vi "IMAQWriteMultiMetadata.vi"(0 "GRMActor in":refnum<class "GenericActor.lvclass">, 5 "Image In":T1, 7 "Keys":string[](array[string]), 9 "Values":dbl[](array[numeric]), 11 "error in (no error)":errorcluster, 12 "precision (6)":i16) -> (4 "GRMActor out":refnum<class "GenericActor.lvclass">, 6 "Image Out":T1, 15 "error out":errorcluster)   [LabVIEW 2020, in "GenericActor.lvlib" / "GenericActor.lvclass"]
uses:
  GenericActor.lvclass
  <vilib>/vision/Image Controls.llb/IMAQ Image.ctl
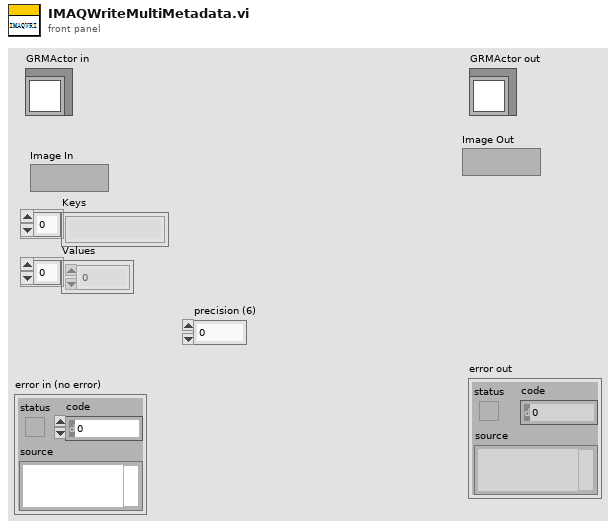
[diagram p1: front panel]
types:
  T1 = typedef "IMAQ Image.ctl" = refnum<image>
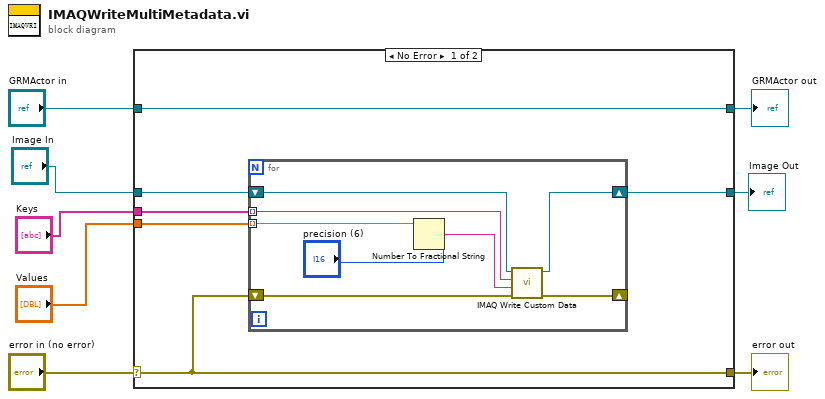
[diagram p0: block diagram]
diagram:
  n1 = case shown="No Error" "error in (no error)" {
    selector: "error in (no error)" -> [w9 w25]
    tunnel: [w9 w25] -> w7
    tunnel: [w14 w24] -> w5
    tunnel: "GRMActor in" -> [w14 w24]
    tunnel: "Image In" -> [w13 w23]
    tunnel: "Keys" -> [w12 _]
    tunnel: "Values" -> [w11 _]
    tunnel: [w10 w23] -> w1
    frame No Error {
      n2 = for {
        tunnel: w12 -> [w17] mode=indexing
        tunnel: w11 -> [w16] mode=indexing
        shift-right: [w21] -> _
        shift-left: w9 -> [w22]
        shift-right: [w19] -> w10
        shift-left: w13 -> [w20]
        n3 = Number To Fractional String(number=w16, precision (6)="precision (6)") -> (F-format string=w18:string)  [unwired: 2 in]
        n4 = call "IMAQ Write Custom Data"("error in (no error)"=w22, "Custom Data In"=w18, "Key"=w17, "Image"=w20) -> ("error out"=w21:errorcluster, "Image Out"=w19:T1)  [unwired: 6 in]
      }
    }
    frame Error {
    }
  }
  "error out" <- w7
  "GRMActor out" <- w5
  "Image Out" <- w1
